vi "test quick start same name  module.vi"() -> ()   [LabVIEW 2017]
uses:
  user.lib/_NEVSTOP/Communicable State Machine(CSM)/Utility/_support/Periodic String Filter Level.ctl
  user.lib/_NEVSTOP/Communicable State Machine(CSM)/Utility/Periodic String Filter Setting.ctl
  ac89a7a7-fb92-48a0-9e52-bad48906b6c3.vi
  user.lib/_NEVSTOP/Communicable State Machine(CSM)/Communicable State Machine.lvlib
  user.lib/_NEVSTOP/Communicable State Machine(CSM)/_Shared/CSM Shared.lvlib
panel:
  out "LogInQ":i32
  out "State History":string
  out "log handling Speed(#/s)":dbl
  out "LogInQ change(#/s)":dbl
  out "Level":T1
  in  "Stop":bool
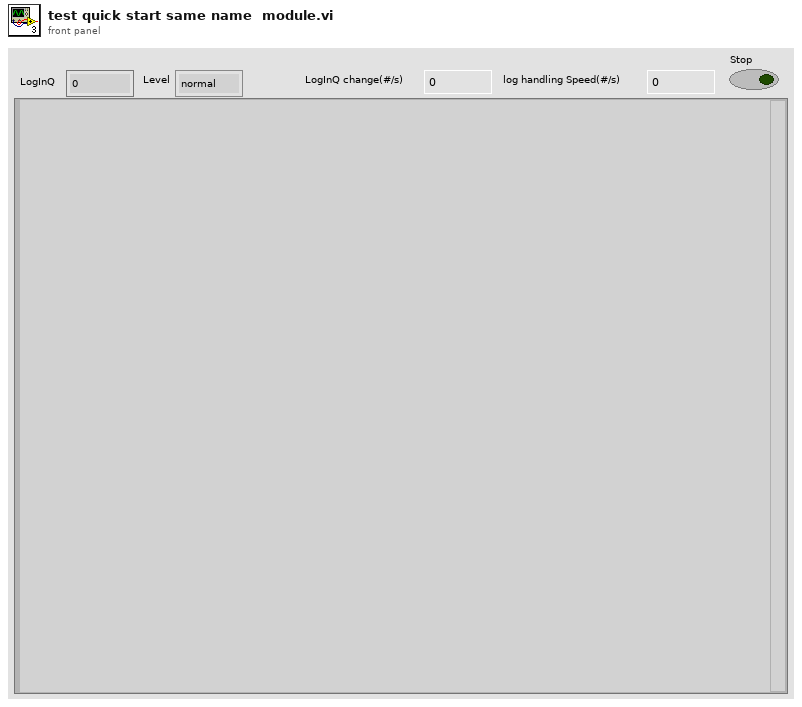
[diagram p1: front panel]
types:
  T1 = typedef "Communicable State Machine.lvlib/Periodic String Filter Level.ctl" = enum16{"normal", "L1", "L2", "L3", "L4"}
  T2 = typedef "Communicable State Machine.lvlib/Periodic String Filter Setting.ctl" = cluster{"threashold(#/s)":dbl, "Check Peroid(s)":dbl}
  T3 = typedef "Communicable State Machine.lvlib/_CSM_GlobalLog_MSG.ctl" = cluster{"Name (\"\" to Use UUID)":string, "Current State":string, "Arguments":string, "Source Message":T4, "Source Module":string, "Complete(T)/Start(F)":bool, "LogType":T5, "Time Stamp":timestamp}
  T4 = typedef "Communicable State Machine.lvlib/_CSM_Response Source Message.ctl" = cluster{"‘State":string, "’Arguments":string, "’Error":errorcluster}
  T5 = typedef "Communicable State Machine.lvlib/_CSM_GlobalLog_MSG_TYPE.ctl" = enum16{"User Log", "State Change", "Status", "Interrupt", "Register", "Unregister", "Error Log", "Module Created", "Module Destroyed"}
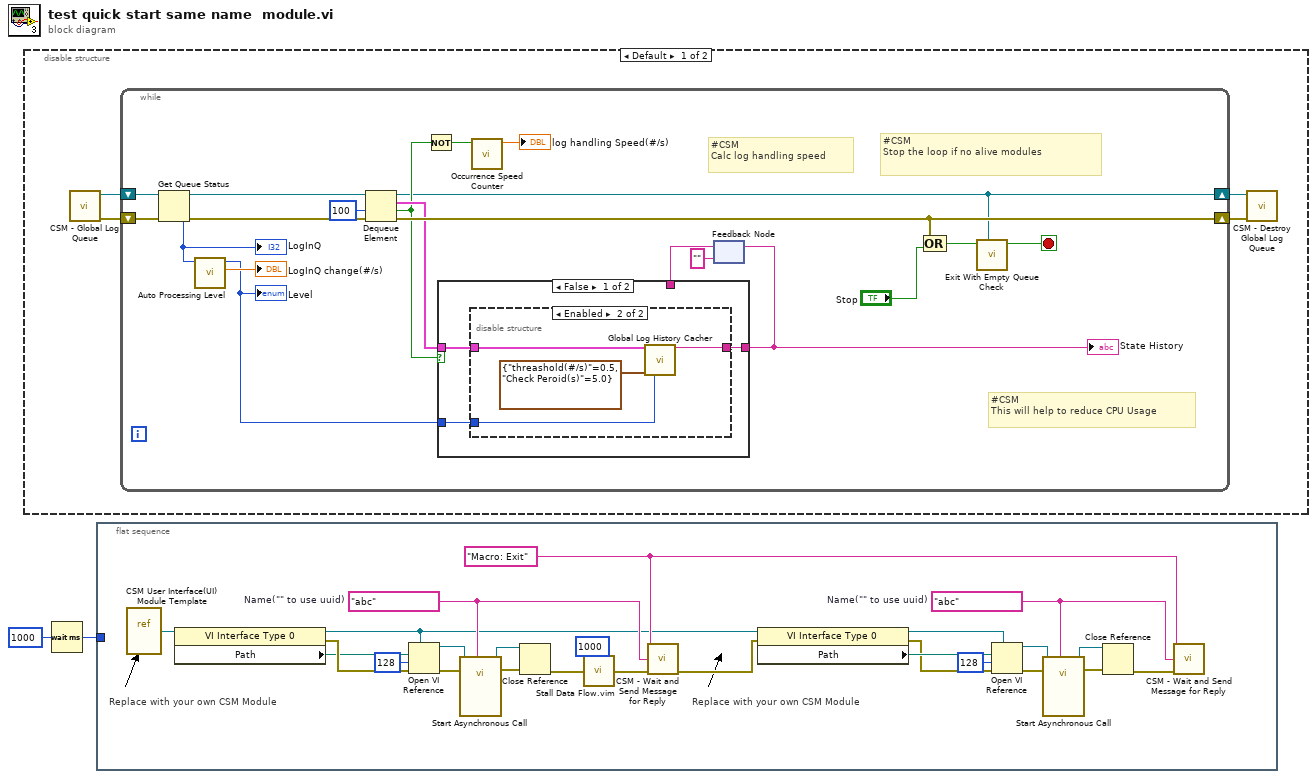
[diagram p0: block diagram]
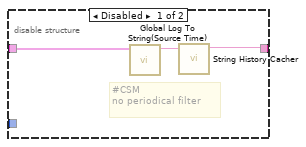
[diagram p2: hidden frame]
diagram:
  n1 = disable-structure shown="Default" {
    frame condition #0 (active) {
      n2 = call "CSM - Global Log Queue.vi"() -> ("error out"=w5:errorcluster, "GlobalEvent Queue"=w3:refnum<queue>)  [unwired: 10 in]
      n3 = while {
        shift-right: [w25] -> w6
        shift-left: w5 -> [w22]
        shift-right: [w13] -> w4
        shift-left: w3 -> [w26]
        stop <- w7 stop-if-true
        # "#CSM\nCalc log handling speed"
        # "#CSM\nStop the loop if no alive modules"
        # "#CSM\nThis will help to reduce CPU Usage"
        n4 = Get Queue Status(queue=w26, error in (no error)=w22) -> (queue out=w24:refnum<queue>, error out=w23:errorcluster, # elements in queue=w10:i32)  [unwired: 1 in, 5 out]
        "LogInQ" <- w10
        n5 = call "Auto Processing Level.vi"("#Left In Q"=w10) -> ("LogInQ Changing Speed (#/s)"=→"LogInQ change(#/s)":dbl, "Level"=w9:T1)  [unwired: 8 in, 1 out]
        "Level" <- w9
        n6 = Dequeue Element(queue=w24, timeout in ms (-1)=100, error in (no error)=w23) -> (queue out=w13:refnum<queue>, element=w21:T3, timed out?=w15:bool, error out=w25:errorcluster)
        n7 = Not(x=w15) -> (.not. x?=w14:bool)
        n8 = call "Occurrence Speed Counter.vi"("Occured? (T)"=w14) -> ("Speed (#/s)"=→"log handling Speed(#/s)":dbl)  [unwired: 8 in, 2 out]
        n9 = feedback #1("" ("String Cache")) -> (w18:string)
        n10 = case shown="False" w15 {
          tunnel: w21 -> [w29 _]
          tunnel: [w28 w37] -> w19
          tunnel: w18 -> [_ w37]
          tunnel: w9 -> [w27 _]
          frame False {
            n11 = disable-structure shown="Enabled" {
              disable-tunnel: w29 -> [w32 w35]
              disable-tunnel: [w30 w36] -> w28
              disable-tunnel: w27 -> [_ w34]
              frame Disabled {
                # "#CSM \nno periodical filter"
                n12 = call "Global Log To String(Source Time).vi"("Log"=w32) -> ("Log String"=w31:string)  [unwired: 9 in]
                n13 = call "String History Cacher.vi"("String"=w31) -> ("String Cache"=w30:string)  [unwired: 10 in]
              }
              frame Enabled {
                n14 = call "Global Log History Cacher.vi"("Cross CSM Data"=w35, "Settings"=T2 {"threashold(#/s)"=0.5, "Check Peroid(s)"=5.0}, "Level (Normal)"=w34) -> ("String Cache"=w36:string)  [unwired: 12 in]
              }
            }
          }
          frame True {
          }
        }
        "State History" <- w19
        n15 = feedback-in #1(w19) -> ()
        n16 = Compound Arithmetic op=OR(w25, "Stop") -> (w12:bool)
        n17 = call "Exit With Empty Queue Check.vi"("Queue"=w13, "Stop"=w12) -> ("Exit"=w7:bool)  [unwired: 8 in, 1 out]
      }
      n18 = call "CSM - Destroy Global Log Queue.vi"("Error In"=w6, "Global Log Queue"=w4) -> ()  [unwired: 9 in, 1 out]
    }
    frame condition #1 {
    }
  }
  n19 = Wait (ms)(milliseconds to wait=u32 1000) -> (millisecond timer value=w1:u32)
  n20 = flat-sequence {
    tunnel: w1 -> [_]
    frame #0 {
      w52 = "abc"  # Name("" to use uuid)
      w41 = "Macro: Exit" ("State")
      w53 = "abc"  # Name("" to use uuid)
      # "Replace with your own CSM Module"
      # "Replace with your own CSM Module"
      n21 = vi-ref "CSM User Interface(UI) Module Template.vi"() -> (w56:refnum<vi>)
      n22 = property class="VI Interface Type 0"(reference=w56) -> (reference out=w40:refnum<vi>, error out=w58:errorcluster, "Path"=w57:path)  [unwired: 1 in]
      n23 = Open VI Reference(type specifier VI Refnum (for type only)=w40, vi path=w57, options=128, error in (no error)=w58) -> (vi reference=w59:refnum<vi>, error out=w55:errorcluster)  [unwired: 2 in]
      n24 = call-by-ref "Start Asynchronous Call"(reference=w59, error in=w55, "Name(\"\" to use uuid)"=w53) -> (reference out=w61:refnum<vi>, error out=w60:errorcluster)  [unwired: 11 in]
      n25 = Close Reference(reference=w61, error in (no error)=w60) -> (error out=w54:errorcluster)
      n26 = call "Stall Data Flow.vim"("value in"=w54, "milliseconds to wait"=u32 1000) -> ("value out"=w39:errorcluster)  [unwired: 1 out]
      n27 = call "CSM - Wait and Send Message for Reply.vi"("State"=w41, "Target Module"=w53, "Error In (No Error)"=w39) -> ("error out"=w42:errorcluster)  [unwired: 10 in, 2 out]
      n28 = property class="VI Interface Type 0"(reference=w40, error in=w42) -> (reference out=w46:refnum<vi>, error out=w48:errorcluster, "Path"=w49:path)
      n29 = Open VI Reference(type specifier VI Refnum (for type only)=w46, vi path=w49, options=128, error in (no error)=w48) -> (vi reference=w47:refnum<vi>, error out=w50:errorcluster)  [unwired: 2 in]
      n30 = call-by-ref "Start Asynchronous Call"(reference=w47, error in=w50, "Name(\"\" to use uuid)"=w52) -> (reference out=w44:refnum<vi>, error out=w45:errorcluster)  [unwired: 11 in]
      n31 = Close Reference(reference=w44, error in (no error)=w45) -> (error out=w51:errorcluster)
      n32 = call "CSM - Wait and Send Message for Reply.vi"("State"=w41, "Target Module"=w52, "Error In (No Error)"=w51) -> ()  [unwired: 10 in, 3 out]
    }
  }
